vi "移动平均.vi"(8 "error in (no error)":errorcluster caption="错误输入（无错误）", 9 "重置":bool, 10 "队列长度":i32=8, 11 "输入数据":dbl) -> (0 "error out":errorcluster, 2 "平均值":dbl, 3 "和":dbl)   [LabVIEW 2011]
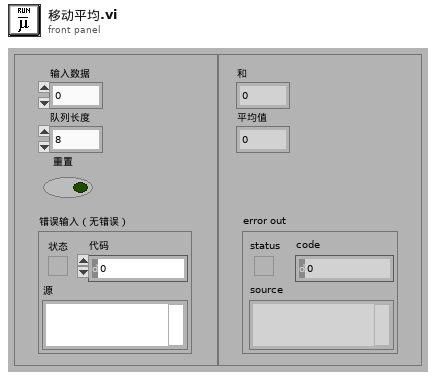
[diagram p1: front panel]
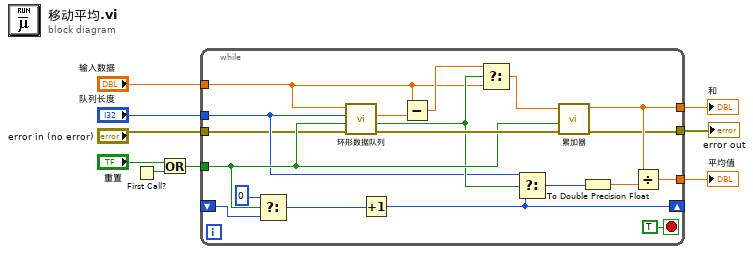
[diagram p0: block diagram]
diagram:
  n1 = First Call?() -> (First Call?: T/F=w5:bool)
  n2 = Or(x="重置", y=w5) -> (x .or. y?=w4:bool)
  n3 = while {
    tunnel: "队列长度" -> [w18]
    tunnel: w4 -> [w24]
    tunnel: [w16] -> w8
    shift-right: [w17] -> _
    shift-left: _ -> [w21]
    tunnel: [w13] -> w7
    tunnel: "输入数据" -> [w12]
    tunnel: "error in (no error)" -> [w11]
    tunnel: [w10] -> w1
    stop <- TRUE stop-if-true
    n4 = Select(t=0 ("队列长度"), s=w24, f=w21) -> (s? t:f=w22:i32)
    n5 = call-poly "环形数据队列.vi"("error in (no error)"=w11, "重置"=w24, "队列长度"=w18, "输入数据"=w12) -> ("error out"=w28:errorcluster, "队列满"=w19:bool, "出队元素"=w27:dbl)  [unwired: 4 in, 1 out]
    n6 = Increment(x=w22) -> (x+1=w17:i32)
    n7 = Subtract(x=w12, y=w27) -> (x-y=w26:dbl)
    n8 = Select(t=w26, s=w19, f=w12) -> (s? t:f=w25:dbl)
    n9 = Select(t=w18, s=w19, f=w17) -> (s? t:f=w15:i32)
    n10 = call-poly "累加器.vi"("error in"=w28, "reset"=w24, "input"=w25) -> ("error out"=w10:errorcluster, "accumulation"=w16:dbl)  [unwired: 7 in]
    n11 = To Double Precision Float(number=w15) -> (double precision float=w14:dbl)
    n12 = Divide(x=w16, y=w14) -> (x/y=w13:dbl)
  }
  "和" <- w8
  "平均值" <- w7
  "error out" <- w1
